vi "Read Window Write Size.vi"(5 "Username":string, 6 "Password":string, 7 "Address":string, 8 "Error In":errorcluster) -> (0 "Error Out":errorcluster)   [LabVIEW 2018, in "Tests.lvlib" / "Channel.lvlib"]
uses:
  Channel.lvlib
  src/Toolkit/Channel/Channel.lvclass/Channel.ctl
  src/Toolkit/Session/Session.lvclass/Session.ctl
  src/Toolkit/SSH/SSH.lvclass/SSH.ctl
  src/Toolkit/Session/Utility/Read Shared Library.vi
  src/Toolkit/SSH/Utility/Read Shared Library.vi
  src/Toolkit/Support/Check Status.vi
  <vilib>/addons/_JKI Toolkits/Caraya/classes/Test/Test.lvclass
  <vilib>/addons/_JKI Toolkits/Caraya/classes/Assert/Assert.lvclass
  src/Toolkit/Channel/Channel.lvclass
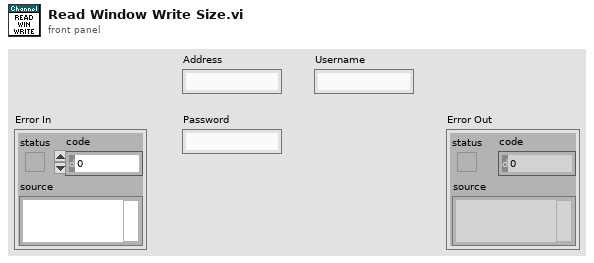
[diagram p1: front panel]
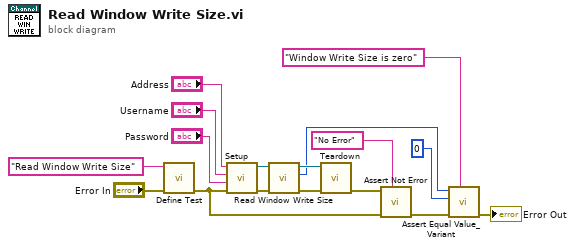
[diagram p0: block diagram]
diagram:
  n1 = call <vilib>:"Define Test.vi"("error in (no error)"="Error In", "Label (VI Title)"="Read Window Write Size") -> ("error out"=w14:errorcluster)  [unwired: 9 in]
  n2 = call "Setup.vi"("Error In"=w14, "Password"="Password", "Username"="Username", "Address"="Address") -> ("Error Out"=w7:errorcluster, "Channel"=w8:refnum<class "Channel.lvclass">)  [unwired: 6 in]
  n3 = call "Read Window Write Size.vi"("Error In"=w7, "Channel In"=w8) -> ("Error Out"=w6:errorcluster, "Write Size"=w3:u32, "Channel Out"=w5:refnum<class "Channel.lvclass">)  [unwired: 7 in]
  n4 = call "Teardown.vi"("Error In"=w6, "Channel"=w5) -> ("Error Out"=w10:errorcluster)  [unwired: 9 in]
  n5 = call <vilib>:"Assert Not Error.vi"("Label"="No Error", "error in (no error)"=w14, "Not Error?"=w10) -> ("error out"=w9:errorcluster)  [unwired: 8 in]
  n6 = call <vilib>:"Assert Equal Value_Variant.vi"("Label"="Window Write Size is zero", "error in (no error)"=w9, "Y"=u32 0 ("Size"), "X"=w3) -> ("error out"=→"Error Out":errorcluster)  [unwired: 7 in]
